vi "launch_vi.vi"(7 "transition_queue":refnum<queue>, 8 "error in (no error)":errorcluster, 10 "data":T1, 11 "vi_reference":variant) -> (0 "error out":errorcluster)   [LabVIEW 2015, in "lv-recipe-machine.lvlib"]
uses:
  lv-recipe-machine.lvlib
  _controls/automatic_vi_variant_data.ctl
  public/_controls/automatic_state.ctl
  public/_controls/transition.ctl
  public/_controls/error.ctl
  public/_controls/vi_reference_type.ctl
  public/_controls/vi_reference_manual_action.ctl
  public/_controls/vi_reference_criteria.ctl
  public/_controls/vi_reference_launch.ctl
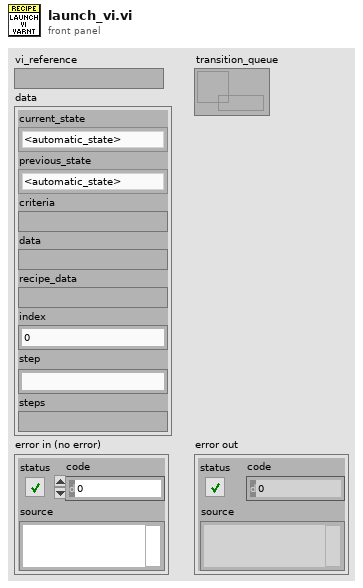
[diagram p1: front panel]
types:
  T1 = typedef "lv-recipe-machine.lvlib/automatic_vi_variant_data.ctl" = cluster{"current_state":T2, "previous_state":T2, "criteria":variant, "data":variant, "recipe_data":variant, "index":i32, "step":string, "steps":variant}
  T2 = typedef "lv-recipe-machine.lvlib/automatic_state.ctl" = enum16{"<automatic_state>", "failed", "idle", "running", "paused", "stopped", "<null>"}
  T3 = typedef "lv-recipe-machine.lvlib/error.ctl" = enum16{"<error>", "bad_command", "command_queue_timeout", "stop_notifier_timeout", "die_command_timeout", "not_in_manual_mode", "not_in_automatic_mode", "not_in_automatic_idle", "not_in_automatic_running", "not_in_automatic_paused", "automatic_step_not_found", "manual_action_not_found", "automatic_not_transition_vi", "transition_step_not_found", "unsupported_vi_type", "<null>"}
  T4 = typedef "lv-recipe-machine.lvlib/vi_reference_type.ctl" = enum16{"<vi_reference_type>", "manual_action", "auto_step", "auto_criteria", "auto_transition", "auto_launcher", "<null>"}
  T5 = typedef "lv-recipe-machine.lvlib/vi_reference_manual_action.ctl" = refnum<vi>
  T6 = typedef "lv-recipe-machine.lvlib/vi_reference_criteria.ctl" = refnum<vi>
  T7 = typedef "lv-recipe-machine.lvlib/vi_reference_launch.ctl" = refnum<vi>
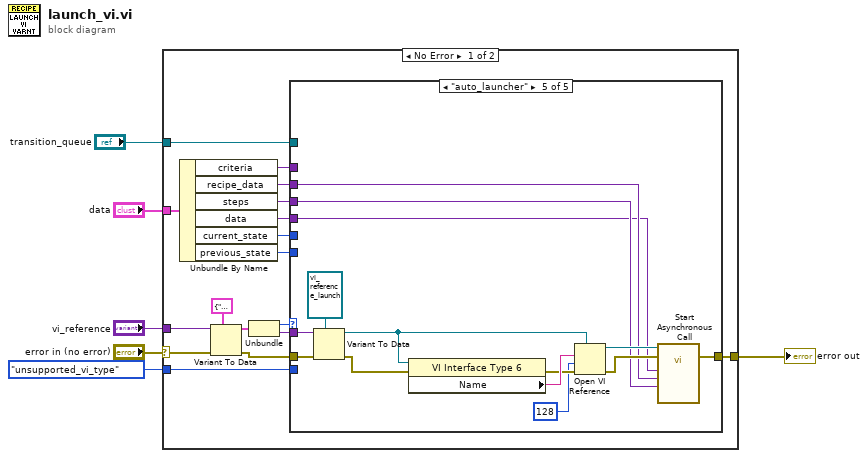
[diagram p0: block diagram]
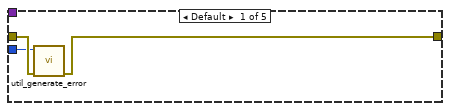
[diagram p2: hidden frame]
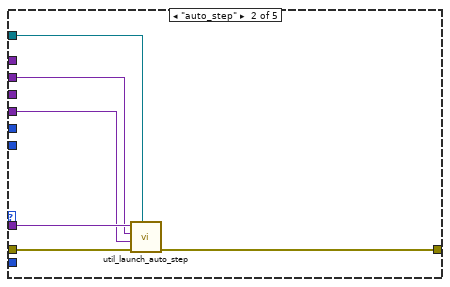
[diagram p3: hidden frame]
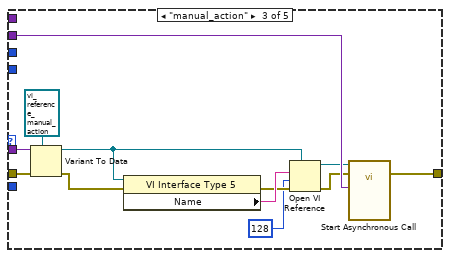
[diagram p4: hidden frame]
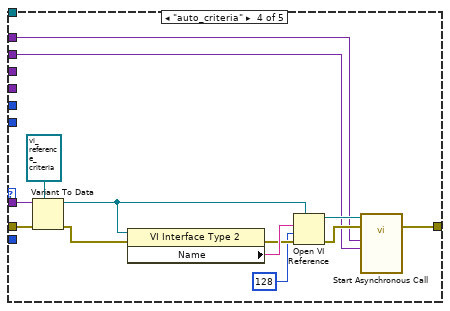
[diagram p5: hidden frame]
diagram:
  n1 = case shown="No Error" "error in (no error)" {
    selector: "error in (no error)" -> [w16 w72]
    tunnel: [w23 w72] -> w5
    tunnel: "vi_reference" -> [w17 _]
    tunnel: "data" -> [w22 _]
    tunnel: error."unsupported_vi_type" ("error") -> [w9 _]
    tunnel: "transition_queue" -> [w7 _]
    frame No Error {
      n2 = Unbundle By Name(w22) -> ("criteria"=w21:variant, "recipe_data"=w20:variant, "steps"=w8:variant, "data"=w19:variant, "current_state"=w11:T2, "previous_state"=w10:T2)
      n3 = Variant To Data(error in=w16, type=cluster{"vi_reference_type":T4, variant} {"vi_reference_type"=enum."<vi_reference_type>", variant}, Variant=w17) -> (data=w15:cluster{"vi_reference_type":T4, variant}, error out=w14:errorcluster)
      n4 = Unbundle(w15) -> ("vi_reference_type"=w12:T4, w13:variant)
      n5 = case shown="\"auto_launcher\"" w12 {
        tunnel: w13 -> [_ w30 w44 w57 w71]
        tunnel: w14 -> [w26 w32 w43 w56 w70]
        tunnel: [w25 w31 w42 w53 w68] -> w23
        tunnel: w11 -> [_ _ _ _ _]
        tunnel: w10 -> [_ _ _ _ _]
        tunnel: w21 -> [_ _ _ w46 _]
        tunnel: w20 -> [_ w29 _ w47 w62]
        tunnel: w19 -> [_ w28 w41 _ w58]
        tunnel: w9 -> [w24 _ _ _ _]
        tunnel: w8 -> [_ _ _ _ w59]
        tunnel: w7 -> [_ w27 _ _ _]
        frame Default {
          n6 = call "util_generate_error.vi"("error in (no error)"=w26, "error"=w24) -> ("error out"=w25:errorcluster)  [unwired: 9 in]
        }
        frame "auto_step" {
          n7 = call "util_launch_auto_step.vi"("transition_queue"=w27, "error in (no error)"=w32, "data"=w28, "recipe_data"=w29, "vi_reference"=w30) -> ("error out"=w31:errorcluster)  [unwired: 6 in]
        }
        frame "manual_action" {
          n8 = Variant To Data(error in=w43, type=T5 refnum ("step_vi_reference"), Variant=w44) -> (data=w34:T5, error out=w33:errorcluster)
          n9 = property class="VI Interface Type 5"(reference=w34, error in=w33) -> (error out=w38:errorcluster, "Name"=w39:string)  [unwired: 1 out]
          n10 = Open VI Reference(type specifier VI Refnum (for type only)=w34, vi path=w39, options=128, error in (no error)=w38) -> (vi reference=w37:T5, error out=w40:errorcluster)  [unwired: 2 in]
          n11 = call-by-ref "Start Asynchronous Call"(reference=w37, error in=w40, "data"=w41) -> (error out=w42:errorcluster)  [unwired: 10 in, 2 out]
        }
        frame "auto_criteria" {
          n12 = Variant To Data(error in=w56, type=T6 refnum ("vi_reference_criteria"), Variant=w57) -> (data=w54:T6, error out=w45:errorcluster)
          n13 = property class="VI Interface Type 2"(reference=w54, error in=w45) -> (error out=w50:errorcluster, "Name"=w51:string)  [unwired: 1 out]
          n14 = Open VI Reference(type specifier VI Refnum (for type only)=w54, vi path=w51, options=128, error in (no error)=w50) -> (vi reference=w49:T6, error out=w52:errorcluster)  [unwired: 2 in]
          n15 = call-by-ref "Start Asynchronous Call"(reference=w49, error in=w52, "recipe_data"=w47, "criteria"=w46) -> (error out=w53:errorcluster)  [unwired: 9 in, 2 out]
        }
        frame "auto_launcher" {
          n16 = Variant To Data(error in=w70, type=T7 refnum, Variant=w71) -> (data=w69:T7, error out=w61:errorcluster)
          n17 = property class="VI Interface Type 6"(reference=w69, error in=w61) -> (error out=w65:errorcluster, "Name"=w66:string)  [unwired: 1 out]
          n18 = Open VI Reference(type specifier VI Refnum (for type only)=w69, vi path=w66, options=128, error in (no error)=w65) -> (vi reference=w64:T7, error out=w67:errorcluster)  [unwired: 2 in]
          n19 = call-by-ref "Start Asynchronous Call"(reference=w64, error in=w67, "steps"=w59, "recipe_data in"=w62, "data"=w58) -> (error out=w68:errorcluster)  [unwired: 8 in, 2 out]
        }
      }
    }
    frame Error {
    }
  }
  "error out" <- w5
